vi "客户端发送.vi"(2 "本机端口":u16, 3 "receive port":u16, 4 "数据输入":string, 5 "IP":string) -> ()   [LabVIEW 2016, in "自动更新.lvlib" / "TCP文件传输系统.lvlib" / "TCP接收文件.lvlib"]
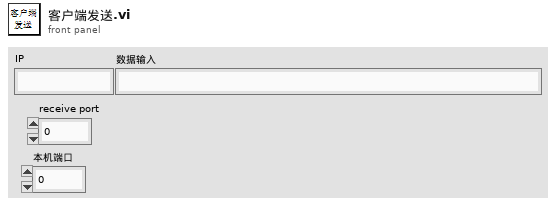
[diagram p1: front panel]
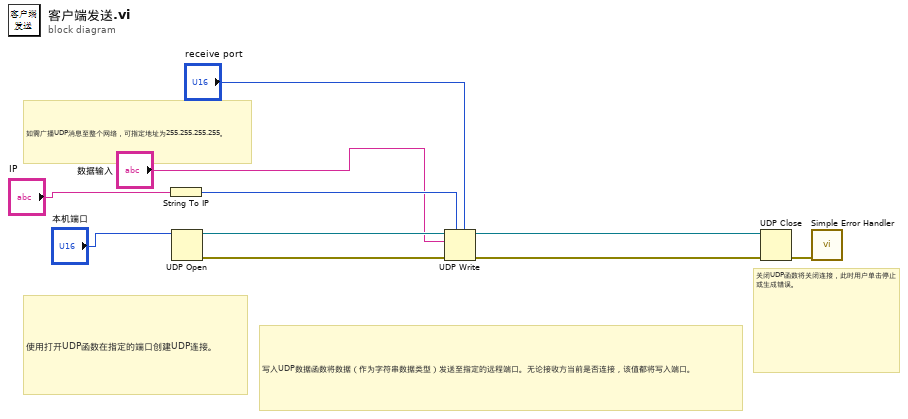
[diagram p0: block diagram]
diagram:
  # "如需广播UDP消息至整个网络，可指定地址为255.255.255.255。"
  # "关闭UDP函数将关闭连接，此时用户单击停止或生成错误。"
  # "写入UDP数据函数将数据（作为字符串数据类型）发送至指定的远程端口。无论接收方当前是否连接，该值都将写入端口。"
  # "使用打开UDP函数在指定的端口创建UDP连接。"
  n1 = String To IP(1:"IP") -> (0:w7:u32)
  n2 = UDP Open(11:"本机端口") -> (port=w6:refnum<k16>, 0:w5:errorcluster)  [unwired: 4 in, 1 out]
  n3 = UDP Write(address=w7, port or service name="receive port", connection ID=w6, data in="数据输入", 8:w5) -> (error out=w9:errorcluster, 3:w10:refnum<k16>)  [unwired: 1 in]
  n4 = UDP Close(connection ID=w10, 8:w9) -> (error out=w8:errorcluster)  [unwired: 1 out]
  n5 = call <vilib>:"Simple Error Handler.vi"("error in (no error)"=w8) -> ()  [unwired: 4 in, 5 out]
